vi "Velocity-Accel and traj adj.vi"(10 "FPS":dbl, 11 "Raw position":dbl[][](array[numeric])) -> (0 "Vel, Accel RMS":dbl[][](array[numeric]), 1 "#Crossings":i32[][](array[numeric]), 2 "Vel, Acc data":dbl[][](array[numeric]), 3 "Velocity-Acceleration graphs":dbl[][](array[numeric]))   [LabVIEW 2020]
uses:
  <vilib>/Analysis/5stat.llb/RMS (DBL).vi
  <vilib>/Analysis/NI_AALPro.lvlib
panel:
  out "Velocity,Acc data":dbl[](array[numeric])
  out "RMS":dbl[](array[numeric])
  out "Velocity, accel Data":dynamicdata[](array[waveform])
  out "Number of crossings Acceleration Y":i32
  out "Number of crossings Velocity Y":i32
  out "Wrist Y (hor) position":dbl[](graph)
  out "Acceleration Y":dbl[](graph)
  out "Velocity Y":dbl[](graph)
  out "Number of crossings Acceleration X":i32
  out "Number of crossings Velocity X":i32
  out "Wrist X (vert) position":dbl[](graph)
  out "Acceleration X":dbl[](graph)
  out "Velocity X":dbl[](graph)
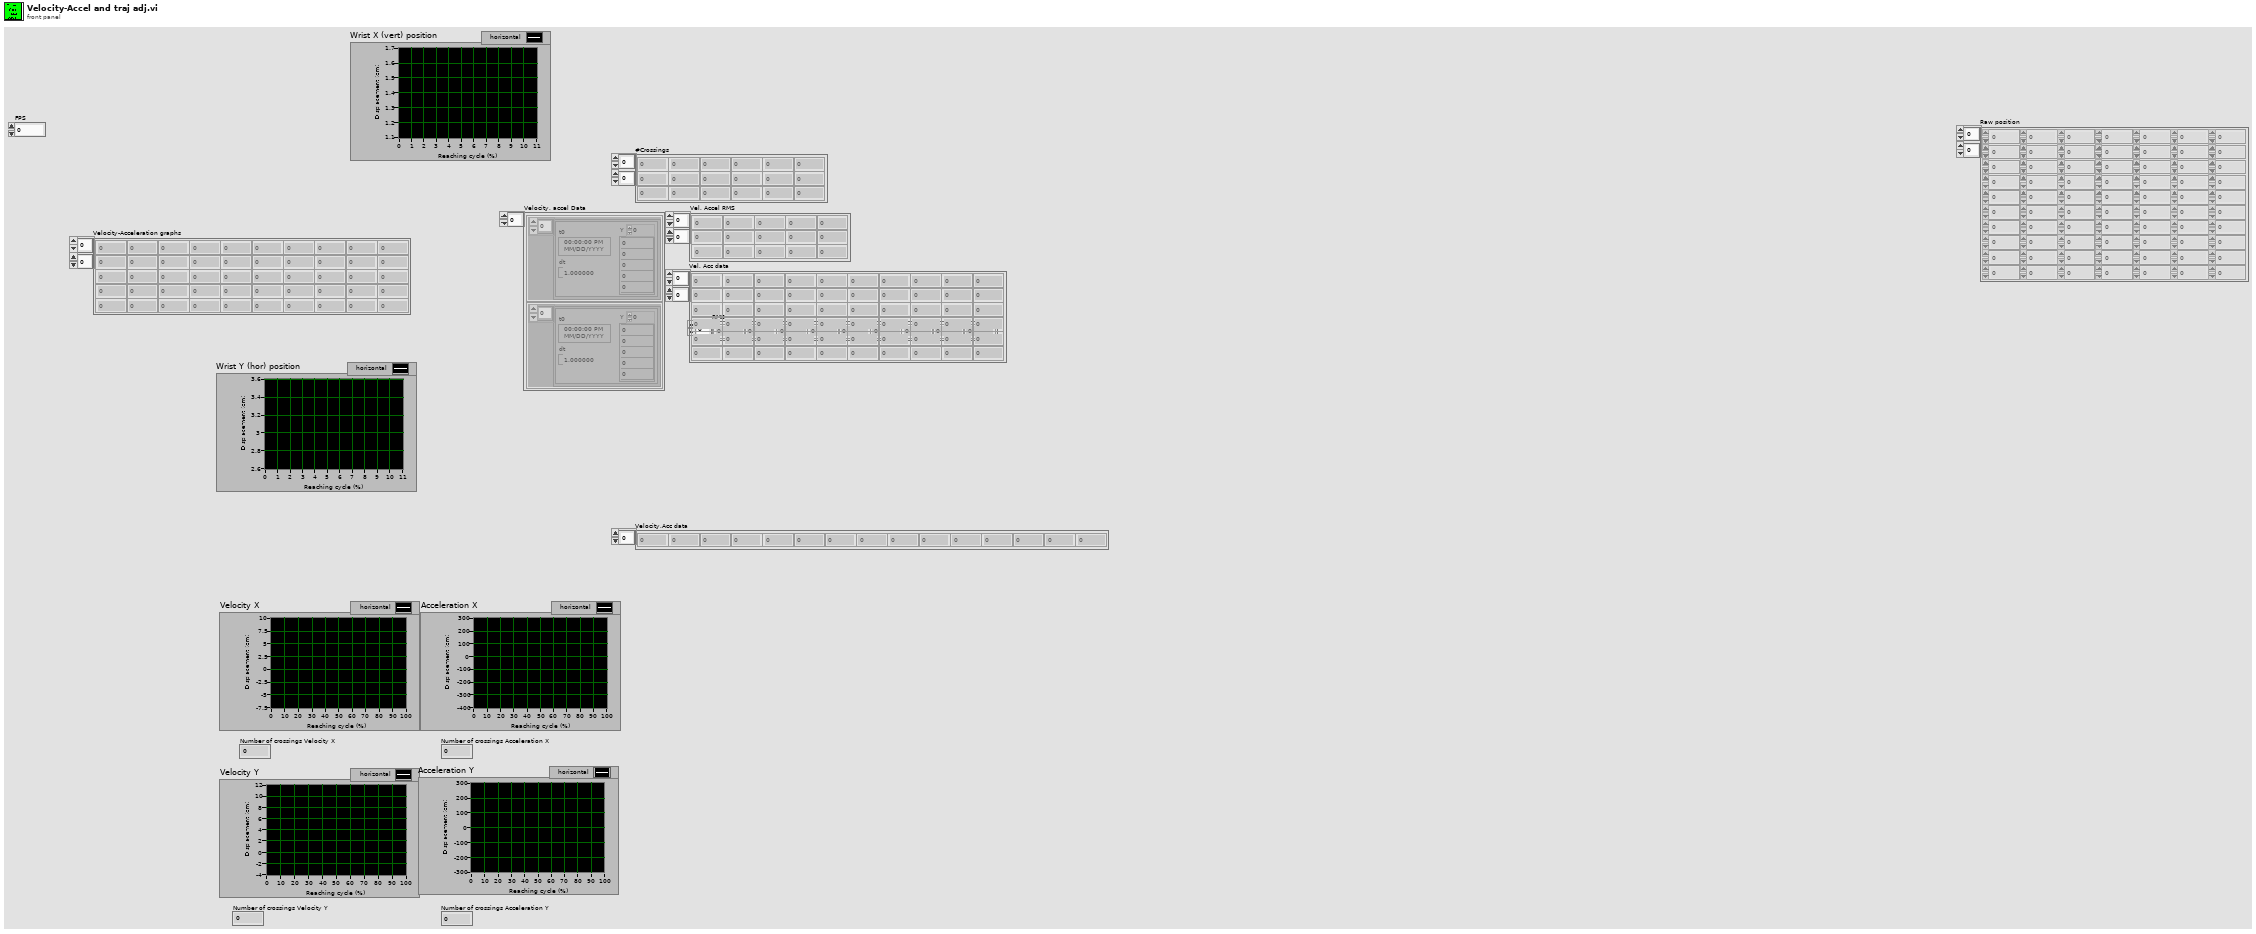
[diagram p1: front panel]
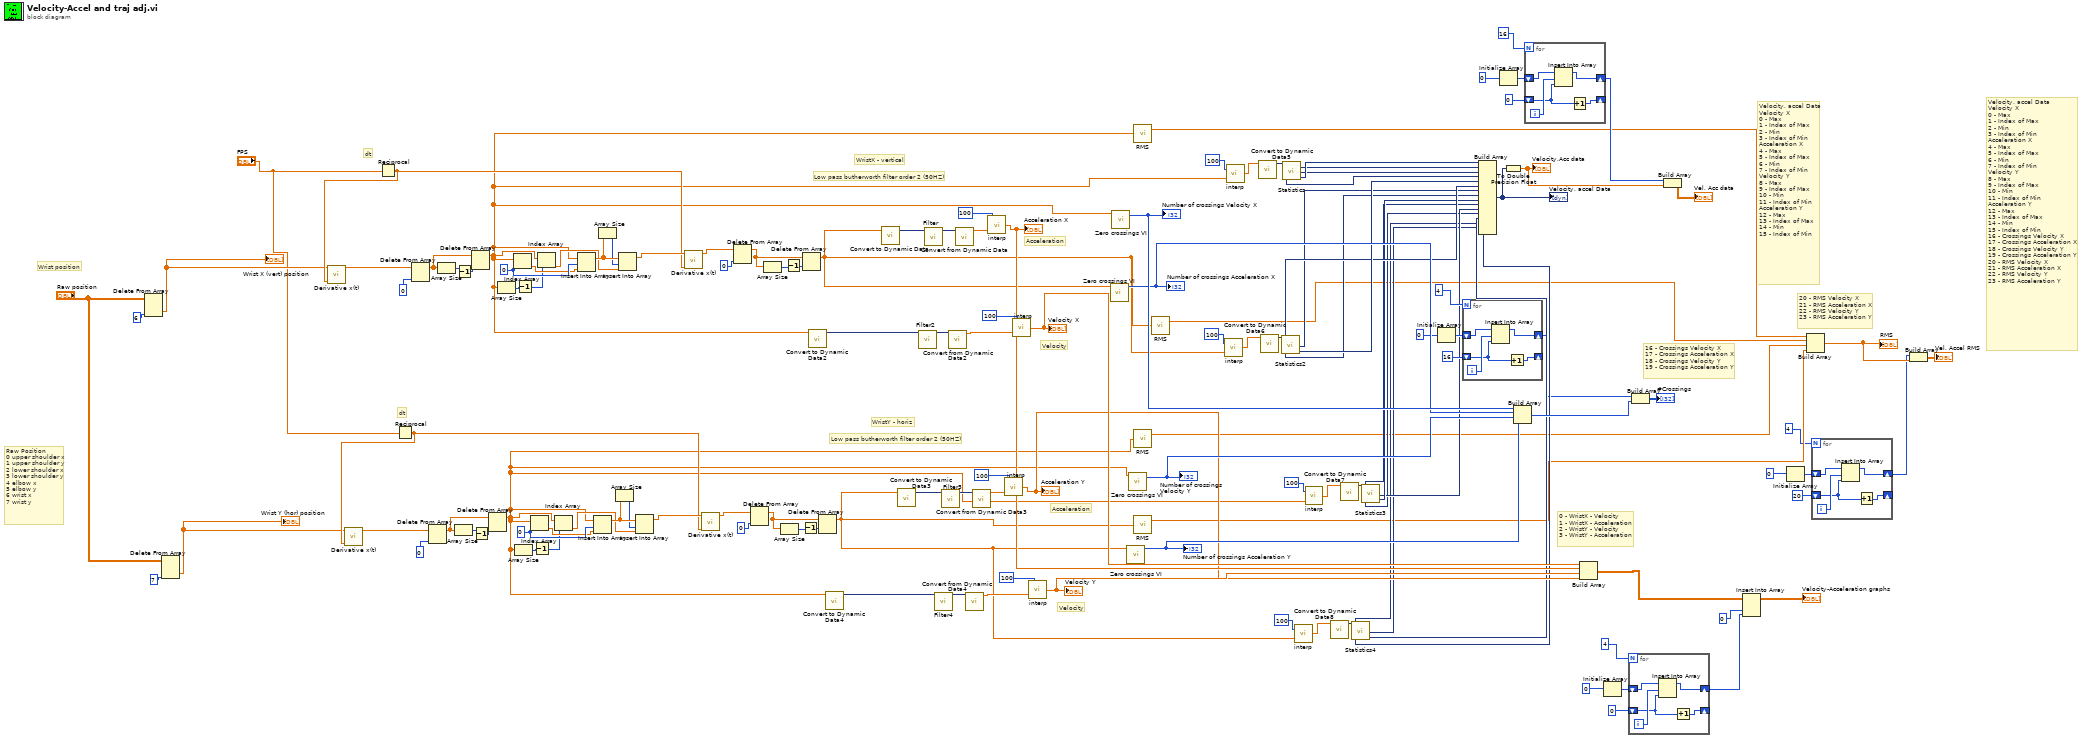
[diagram p0: block diagram]
diagram:
  w102 = 0
  w129 = 0
  # "Velocity, accel Data\nVelocity X\n0 - Max\n1 - Index of Max\n2 - Min\n3 - Index of Min\nAcceleration X\n4 - Max\n5 - Index of Max\n6 - Min\n7 - Index of Min\nVelocity Y\n8 - Max\n9 - Index of Max\n10 - Min\n11 - Index of Min\nAcceleration Y\n12 - Max\n13 - Index of Max\n14 - Min\n15 - Index of Min\n16 - Crossings Velocity X\n17 - Crossings Acceleration X\n18 - Crossings Velocity Y\n19 - Crossings Acceleration Y\n20 - RMS Velocity X\n21 - RMS Acceleration X\n22 - RMS Velocity Y\n23 - RMS Acceleration Y"
  # "20 - RMS Velocity X\n21 - RMS Acceleration X\n22 - RMS Velocity Y\n23 - RMS Acceleration Y"
  # "Velocity, accel Data\nVelocity X\n0 - Max\n1 - Index of Max\n2 - Min\n3 - Index of Min\nAcceleration X\n4 - Max\n5 - Index of Max\n6 - Min\n7 - Index of Min\nVelocity Y\n8 - Max\n9 - Index of Max\n10 - Min\n11 - Index of Min\nAcceleration Y\n12 - Max\n13 - Index of Max\n14 - Min\n15 - Index of Min"
  # "Acceleration"
  # "Acceleration"
  # "dt"
  # "16 - Crossings Velocity X\n17 - Crossings Acceleration X\n18 - Crossings Velocity Y\n19 - Crossings Acceleration Y"
  # "Low pass butherworth filter order 2 (50HZ)"
  # "Velocity"
  # "WristY - horiz"
  # "Raw Position\n0 upper shoulder x\n1 upper shoulder y\n2 lower shoulder x\n3 lower shoulder y\n4 elbow x\n5 elbow y\n6 wrist x\n7 wrist y"
  # "dt"
  # "0 - WristX - Velocity\n1 - WristX - Acceleration\n2 - WristY - Velocity\n3 - WristY - Acceleration"
  # "Low pass butherworth filter order 2 (50HZ)"
  # "Velocity"
  # "WristX - vertical"
  # "Wrist position"
  n1 = Delete From Array(array="Raw position", index (col)=6) -> (deleted portion=w74:dbl[])  [unwired: 2 in, 1 out]
  "Wrist X (vert) position" <- w74
  n2 = Delete From Array(array="Raw position", index (col)=7) -> (deleted portion=w73:dbl[])  [unwired: 2 in, 1 out]
  "Wrist Y (hor) position" <- w73
  n3 = Reciprocal(x="FPS") -> (1/x=w108:dbl)
  n4 = call <vilib>:"Derivative x(t).vi"("dt"=w108, "X"=w74) -> ("dX/dt"=w66:dbl[])  [unwired: 8 in, 1 out]
  n5 = Reciprocal(x="FPS") -> (1/x=w80:dbl)
  n6 = call <vilib>:"Derivative x(t).vi"("dt"=w80, "X"=w73) -> ("dX/dt"=w89:dbl[])  [unwired: 8 in, 1 out]
  n7 = Delete From Array(array=w66, index=0) -> (array with subset deleted=w130:dbl[])  [unwired: 1 in, 1 out]
  n8 = Delete From Array(array=w89, index=0) -> (array with subset deleted=w103:dbl[])  [unwired: 1 in, 1 out]
  n9 = Array Size(array=w130) -> (size(s)=w116:i32)
  n10 = Array Size(array=w103) -> (size(s)=w88:i32)
  n11 = Decrement(x=w116) -> (x-1=w115:i32)
  n12 = Delete From Array(array=w130, index=w115) -> (array with subset deleted=w26:dbl[])  [unwired: 1 in, 1 out]
  n13 = Decrement(x=w88) -> (x-1=w87:i32)
  n14 = Delete From Array(array=w103, index=w87) -> (array with subset deleted=w24:dbl[])  [unwired: 1 in, 1 out]
  n15 = Array Size(array=w26) -> (size(s)=w124:i32)
  n16 = Index Array(array=w26, index=w129) -> (element=w128:dbl)
  n17 = Array Size(array=w24) -> (size(s)=w97:i32)
  n18 = Decrement(x=w124) -> (x-1=w123:i32)
  n19 = Index Array(array=w24, index=w102) -> (element=w101:dbl)
  n20 = Decrement(x=w97) -> (x-1=w96:i32)
  n21 = Index Array(array=w26, index=w123) -> (element=w125:dbl)
  n22 = Index Array(array=w24, index=w96) -> (element=w98:dbl)
  n23 = Insert Into Array(array=w26, index=w129, new element=w128) -> (w127:dbl[])
  n24 = Insert Into Array(array=w24, index=w102, new element=w101) -> (w100:dbl[])
  n25 = Array Size(array=w127) -> (size(s)=w126:i32)
  n26 = Array Size(array=w100) -> (size(s)=w99:i32)
  n27 = Insert Into Array(array=w127, index=w126, new element=w125) -> (w122:dbl[])
  n28 = Insert Into Array(array=w100, index=w99, new element=w98) -> (w95:dbl[])
  n29 = call <vilib>:"Derivative x(t).vi"("dt"=w108, "X"=w122) -> ("dX/dt"=w120:dbl[])  [unwired: 8 in, 1 out]
  n30 = call <vilib>:"Derivative x(t).vi"("dt"=w80, "X"=w95) -> ("dX/dt"=w93:dbl[])  [unwired: 8 in, 1 out]
  n31 = Delete From Array(array=w120, index=0) -> (array with subset deleted=w119:dbl[])  [unwired: 1 in, 1 out]
  n32 = Delete From Array(array=w93, index=0) -> (array with subset deleted=w92:dbl[])  [unwired: 1 in, 1 out]
  n33 = Array Size(array=w119) -> (size(s)=w118:i32)
  n34 = Array Size(array=w92) -> (size(s)=w91:i32)
  n35 = Decrement(x=w118) -> (x-1=w117:i32)
  n36 = Decrement(x=w91) -> (x-1=w90:i32)
  n37 = Delete From Array(array=w119, index=w117) -> (array with subset deleted=w25:dbl[])  [unwired: 1 in, 1 out]
  n38 = call "Convert to Dynamic Data2"("Array"=w26) -> ("Dynamic Data Type"=w111:dynamicdata)  [unwired: 3 in]
  n39 = Delete From Array(array=w92, index=w90) -> (array with subset deleted=w23:dbl[])  [unwired: 1 in, 1 out]
  n40 = call "Convert to Dynamic Data4"("Array"=w24) -> ("Dynamic Data Type"=w83:dynamicdata)  [unwired: 3 in]
  n41 = call "Convert to Dynamic Data"("Array"=w25) -> ("Dynamic Data Type"=w114:dynamicdata)  [unwired: 3 in]
  n42 = call "Convert to Dynamic Data3"("Array"=w23) -> ("Dynamic Data Type"=w86:dynamicdata)  [unwired: 3 in]
  n43 = call "Filter2"("Signal"=w111) -> ("Filtered Signal"=w110:dynamicdata)  [unwired: 9 in, 1 out]
  n44 = call "Filter"("Signal"=w114) -> ("Filtered Signal"=w113:dynamicdata)  [unwired: 9 in, 1 out]
  n45 = call "Filter4"("Signal"=w83) -> ("Filtered Signal"=w82:dynamicdata)  [unwired: 9 in, 1 out]
  n46 = call "Filter3"("Signal"=w86) -> ("Filtered Signal"=w85:dynamicdata)  [unwired: 9 in, 1 out]
  n47 = call "Convert from Dynamic Data2"("Dynamic Data Type"=w110) -> ("Array"=w109:dbl[])  [unwired: 3 in]
  n48 = call "Convert from Dynamic Data"("Dynamic Data Type"=w113) -> ("Array"=w112:dbl[])  [unwired: 3 in]
  n49 = call "Convert from Dynamic Data4"("Dynamic Data Type"=w82) -> ("Array"=w81:dbl[])  [unwired: 3 in]
  n50 = call "Convert from Dynamic Data3"("Dynamic Data Type"=w85) -> ("Array"=w84:dbl[])  [unwired: 3 in]
  n51 = call "interp.vi"("first subarray"=w112, "nFRAMES"=100) -> ("emgInterp"=w64:dbl[])
  "Acceleration X" <- w64
  n52 = call "interp.vi"("first subarray"=w84, "nFRAMES"=100) -> ("emgInterp"=w62:dbl[])
  "Acceleration Y" <- w62
  n53 = call "interp.vi"("first subarray"=w109, "nFRAMES"=100) -> ("emgInterp"=w65:dbl[])
  "Velocity X" <- w65
  n54 = call "interp.vi"("first subarray"=w81, "nFRAMES"=100) -> ("emgInterp"=w63:dbl[])
  "Velocity Y" <- w63
  n55 = call "Zero crossings VI.vi"("Derivate"=w25) -> ("Number of crossings"=w77:i32)  [unwired: 10 in]
  "Number of crossings Acceleration X" <- w77
  n56 = call "Zero crossings VI.vi"("Derivate"=w26) -> ("Number of crossings"=w78:i32)  [unwired: 10 in]
  "Number of crossings Velocity X" <- w78
  n57 = call "Zero crossings VI.vi"("Derivate"=w23) -> ("Number of crossings"=w75:i32)  [unwired: 10 in]
  "Number of crossings Acceleration Y" <- w75
  n58 = call "Zero crossings VI.vi"("Derivate"=w24) -> ("Number of crossings"=w76:i32)  [unwired: 10 in]
  "Number of crossings Velocity Y" <- w76
  n59 = call-poly <vilib>:"RMS.vi"("X"=w26) -> ("rms value"=w22:dbl)  [unwired: 1 out]
  n60 = call-poly <vilib>:"RMS.vi"("X"=w24) -> ("rms value"=w20:dbl)  [unwired: 1 out]
  n61 = call-poly <vilib>:"RMS.vi"("X"=w23) -> ("rms value"=w19:dbl)  [unwired: 1 out]
  n62 = call-poly <vilib>:"RMS.vi"("X"=w25) -> ("rms value"=w21:dbl)  [unwired: 1 out]
  n63 = call "interp.vi"("first subarray"=w25, "nFRAMES"=100) -> ("emgInterp"=w54:dbl[])
  n64 = call "interp.vi"("first subarray"=w26, "nFRAMES"=100) -> ("emgInterp"=w10:dbl[])
  n65 = call "Convert to Dynamic Data5"("Array"=w10) -> ("Dynamic Data Type"=w9:dynamicdata)  [unwired: 3 in]
  n66 = call "Convert to Dynamic Data6"("Array"=w54) -> ("Dynamic Data Type"=w55:dynamicdata)  [unwired: 3 in]
  n67 = call "Statistics2"("Signals"=w55) -> ("Index of Max"=w52:dynamicdata, "Index of Min"=w50:dynamicdata, "Minimum"=w51:dynamicdata, "Maximum"=w53:dynamicdata)  [unwired: 22 in, 1 out]
  n68 = call "Statistics"("Signals"=w9) -> ("Index of Max"=w59:dynamicdata, "Index of Min"=w57:dynamicdata, "Minimum"=w58:dynamicdata, "Maximum"=w60:dynamicdata)  [unwired: 22 in, 1 out]
  n69 = call "interp.vi"("first subarray"=w23, "nFRAMES"=100) -> ("emgInterp"=w40:dbl[])
  n70 = call "interp.vi"("first subarray"=w24, "nFRAMES"=100) -> ("emgInterp"=w47:dbl[])
  n71 = call "Convert to Dynamic Data8"("Array"=w40) -> ("Dynamic Data Type"=w41:dynamicdata)  [unwired: 3 in]
  n72 = call "Convert to Dynamic Data7"("Array"=w47) -> ("Dynamic Data Type"=w48:dynamicdata)  [unwired: 3 in]
  n73 = call "Statistics4"("Signals"=w41) -> ("Index of Max"=w38:dynamicdata, "Index of Min"=w36:dynamicdata, "Minimum"=w37:dynamicdata, "Maximum"=w39:dynamicdata)  [unwired: 22 in, 1 out]
  n74 = call "Statistics3"("Signals"=w48) -> ("Index of Max"=w45:dynamicdata, "Index of Min"=w43:dynamicdata, "Minimum"=w44:dynamicdata, "Maximum"=w46:dynamicdata)  [unwired: 22 in, 1 out]
  n75 = Initialize Array(0) -> (w70:i32[])  [unwired: 1 in]
  n76 = for {
    N: 4 -> [_]
    shift-right: [w137] -> w17
    shift-left: w70 -> [w138]
    shift-right: [w135] -> _
    shift-left: 16 -> [w136]
    i -> [w139]
    n77 = Insert Into Array(array=w138, index=w139, new element=w136) -> (w137:i32[])
    n78 = Increment(x=w136) -> (x+1=w135:i32)
  }
  n79 = Build Array(w60, w59, w58, w57, w53, w52, w51, w50, w46, w45, w44, w43, w39, w38, w37, w36) -> (w8:dynamicdata[])
  "Velocity, accel Data" <- w8
  n80 = Initialize Array(0) -> (w33:i32[])  [unwired: 1 in]
  n81 = To Double Precision Float(number=w8) -> (double precision float=w7:dbl[])
  "Velocity,Acc data" <- w7
  n82 = Build Array(w78, w77, w76, w75) -> (w68:i32[])
  n83 = for {
    N: 16 -> [_]
    shift-right: [w142] -> w31
    shift-left: w33 -> [w143]
    shift-right: [w140] -> _
    shift-left: 0 -> [w141]
    i -> [w144]
    n84 = Insert Into Array(array=w143, index=w144, new element=w141) -> (w142:i32[])
    n85 = Increment(x=w141) -> (x+1=w140:i32)
  }
  n86 = Build Array(w65, w64, w63, w62) -> (w29:dbl[][])
  n87 = Initialize Array(0) -> (w4:i32[])  [unwired: 1 in]
  n88 = for {
    N: 4 -> [_]
    shift-right: [w147] -> w2
    shift-left: w4 -> [w148]
    shift-right: [w145] -> _
    shift-left: 0 -> [w146]
    i -> [w149]
    n89 = Insert Into Array(array=w148, index=w149, new element=w146) -> (w147:i32[])
    n90 = Increment(x=w146) -> (x+1=w145:i32)
  }
  n91 = Build Array(w17, w68) -> (→"#Crossings":i32[][])
  n92 = Build Array(w31, w7) -> (→"Vel, Acc data":dbl[][])
  n93 = Insert Into Array(array=w29, index (col)=0, new element=w2) -> (→"Velocity-Acceleration graphs":dbl[][])  [unwired: 1 in]
  n94 = Initialize Array(0) -> (w13:i32[])  [unwired: 1 in]
  n95 = Build Array(w22, w21, w20, w19) -> (w18:dbl[])
  "RMS" <- w18
  n96 = for {
    N: 4 -> [_]
    shift-right: [w152] -> w11
    shift-left: w13 -> [w153]
    shift-right: [w150] -> _
    shift-left: 20 -> [w151]
    i -> [w154]
    n97 = Insert Into Array(array=w153, index=w154, new element=w151) -> (w152:i32[])
    n98 = Increment(x=w151) -> (x+1=w150:i32)
  }
  n99 = Build Array(w11, w18) -> (→"Vel, Accel RMS":dbl[][])
